vi "Signaling Events.vi"(0 "phase voltage spectra":T2(array[cluster]), 1 "signaling frequency (216.66 Hz)":dbl=216.66, 2 "reset? (F)":bool, 5 "current spectra":T2(array[cluster]), 7 "signaling voltage event settings":T5={"detection threshold [%]"=0.3, "start logical 1 length [s]"=2.99, "start logical 0 length [s]"=2.33, "maximum event length [s]"=64.0}, 9 "system info in":refnum<class "EP System Info.lvclass">, 11 "error in (no error)":errorcluster, 12 "timestamp":timestamp, 13 "interval length [s]":dbl=0.2) -> (4 "signaling voltage events":T4(array[cluster]), 10 "system info out":refnum<class "EP System Info.lvclass">, 15 "error out":errorcluster)   [LabVIEW 2014, in "NI_EP_Power Quality.lvlib"]
doc: "Detects signaling voltage events in a voltage spectrum.\n\nThis VI supports measuring single-bus single-line or multiple-bus single-line systems."
uses:
  <vilib>/addons/Electrical Power/PQ/NI_EP_Power Quality.lvlib
  <vilib>/addons/Electrical Power/PQ/Common/Controls/ep_AI Data Channel.ctl
  <vilib>/addons/Electrical Power/PQ/Common/Controls/ep_Phase.ctl
  <vilib>/addons/Electrical Power/PQ/Common/Classes/System Info/EP System Info.lvclass
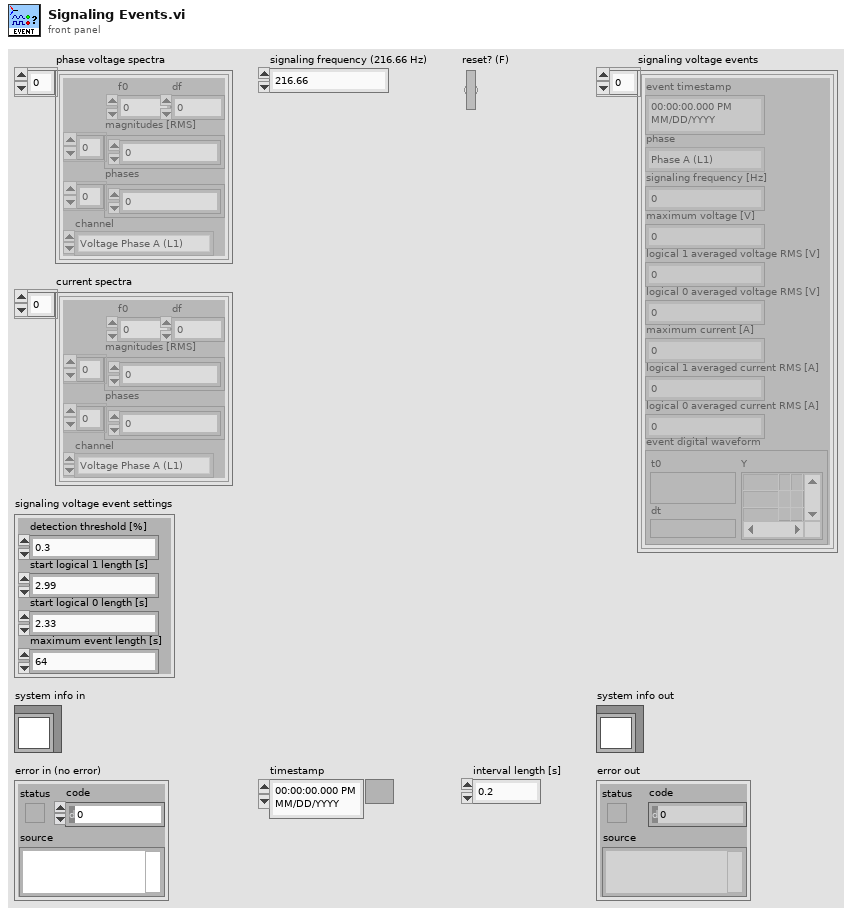
[diagram p1: front panel]
types:
  T1 = typedef "NI_EP_Power Quality.lvlib/ep_AI Data Channel.ctl" = enum16{"Voltage Phase A (L1)", "Voltage Phase B (L2)", "Voltage Phase C (L3)", "Voltage Phase N (Neutral)", "Current Phase A (L1)", "Current Phase B (L2)", "Current Phase C (L3)", "Current Phase N (Neutral)"}
  T2 = cluster{"f0":dbl, "df":dbl, "magnitudes [RMS]":dbl[], "phases":dbl[], "channel":T1}[]
  T3 = typedef "NI_EP_Power Quality.lvlib/ep_Phase.ctl" = enum16{"Phase A (L1)", "Phase B (L2)", "Phase C (L3)", "Phase N", "~3 Phases"}
  T4 = cluster{"event timestamp":timestamp, "phase":T3, "signaling frequency [Hz]":dbl, "maximum voltage [V]":dbl, "logical 1 averaged voltage RMS [V]":dbl, "logical 0 averaged voltage RMS [V]":dbl, "maximum current [A]":dbl, "logical 1 averaged current RMS [A]":dbl, "logical 0 averaged current RMS [A]":dbl, "event digital waveform":digitalwaveform}[]
  T5 = cluster{"detection threshold [%]":dbl, "start logical 1 length [s]":dbl, "start logical 0 length [s]":dbl, "maximum event length [s]":dbl}
  T6 = cluster{"f0":dbl, "df":dbl, "magnitudes [RMS]":dbl[], "phases":dbl[], "channel":T1}
  T7 = cluster{"event time":timestamp, "phase":T3, "signaling frequency [Hz]":dbl, "event voltage max. [V]":dbl, "event voltage log. 1 [V]":dbl, "event voltage log. 0 [V]":dbl, "event current max. [A]":dbl, "event current log. 1 [A]":dbl, "event current log. 0 [A]":dbl, "event digital waveform":digitalwaveform}
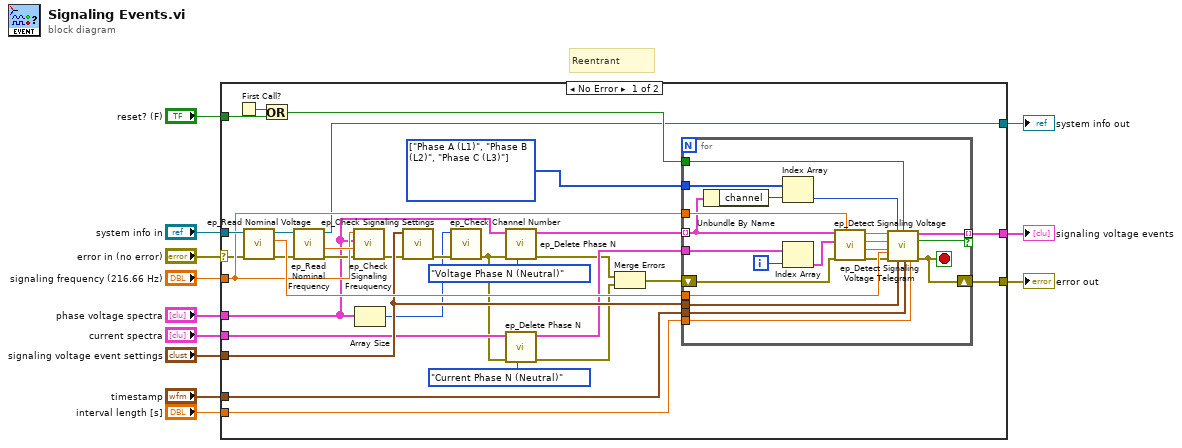
[diagram p0: block diagram]
diagram:
  # "Reentrant"
  n1 = case shown="No Error" "error in (no error)" {
    selector: "error in (no error)" -> [w32 w65]
    tunnel: "system info in" -> [w43 w66]
    tunnel: "current spectra" -> [w19 _]
    tunnel: [w22 w66] -> w10
    tunnel: "timestamp" -> [w20 _]
    tunnel: "interval length [s]" -> [w39 _]
    tunnel: "reset? (F)" -> [w37 _]
    tunnel: "phase voltage spectra" -> [w23 _]
    tunnel: "signaling frequency (216.66 Hz)" -> [w34 _]
    tunnel: [w29 w65] -> w4
    tunnel: "signaling voltage event settings" -> [w33 _]
    tunnel: [w28 _] -> w1
    frame No Error {
      w27 = T3[] [enum."Phase A (L1)", enum."Phase B (L2)", enum."Phase C (L3)"] items=["Phase A (L1)", "Phase B (L2)", "Phase C (L3)", "Phase N", "~3 Phases"]
      n2 = First Call?() -> (First Call?: T/F=w38:bool)
      n3 = call <vilib>:"ep_Read Nominal Voltage.vi"("error in (no error)"=w32, "system info in"=w43) -> ("error out"=w40:errorcluster, "nominal voltage [V]"=w42:dbl, "system info out"=w41:refnum<class "EP System Info.lvclass">)  [unwired: 7 in]
      n4 = Or(x=w38, y=w37) -> (x .or. y?=w36:bool)
      n5 = call <vilib>:"ep_Read Nominal Frequency.vi"("error in (no error)"=w40, "system info in"=w41) -> ("error out"=w31:errorcluster, "nominal frequency value"=w35:dbl, "system info out"=w22:refnum<class "EP System Info.lvclass">)  [unwired: 6 in, 1 out]
      n6 = call <vilib>:"ep_Check Signaling Freuquency.vi"("error in (no error)"=w31, "nominal frequency value"=w35, "phase voltage spectra"=w23, "signaling frequency [Hz]"=w34) -> ("error out"=w30:errorcluster)  [unwired: 7 in]
      n7 = Array Size(array=w23) -> (size(s)=w24:i32)
      n8 = call <vilib>:"ep_Check Signaling Settings.vi"("error in (no error)"=w30, "signaling voltage event settings"=w33) -> ("error out"=w25:errorcluster)  [unwired: 9 in]
      n9 = call <vilib>:"ep_Check Channel Number.vi"("channel number"=w24, "error in (no error)"=w25) -> ("error out"=w18:errorcluster)  [unwired: 13 in]
      n10 = call <vilib>:"ep_Delete Phase N.vi"("channel"=ep_AI_Data_Channel."Voltage Phase N (Neutral)", "error in (no error)"=w18, "spectra in"=w23) -> ("error out"=w14:errorcluster, "spectra out"=w26:T2)  [unwired: 7 in]
      n11 = call <vilib>:"ep_Delete Phase N.vi"("channel"=ep_AI_Data_Channel."Current Phase N (Neutral)", "error in (no error)"=w18, "spectra in"=w19) -> ("error out"=w13:errorcluster, "spectra out"=w16:T2)  [unwired: 7 in]
      n12 = Merge Errors(w14, w13) -> (w15:errorcluster)
      n13 = for {
        tunnel: w42 -> [w64]
        tunnel: w20 -> [w63]
        tunnel: w39 -> [w62]
        tunnel: w36 -> [w61]
        tunnel: w34 -> [w60]
        tunnel: w33 -> [w59]
        tunnel: [w58] -> w28 mode=indexing if=w50
        tunnel: w16 -> [w56]
        tunnel: w26 -> [w47] mode=indexing
        shift-right: [w48] -> w29
        shift-left: w15 -> [w57]
        tunnel: w27 -> [w46]
        i -> [w49]
        stop <- w48 stop-if-true
        n14 = Unbundle By Name(w47) -> ("channel"=w45:T1)
        n15 = Index Array(array=w46, index=w45) -> (element=w44:T3)
        n16 = Index Array(array=w56, index=w49) -> (element=w55:T6)
        n17 = call <vilib>:"ep_Detect Signaling Voltage.vi"("signaling frequency"=w60, "error in (no error)"=w57, "current spectrum (5Hz step)"=w55, "voltage spectrum (5Hz step)"=w47) -> ("error out"=w51:errorcluster, "detected signaling frequency [Hz]"=w52:dbl, "signaling current RMS [A]"=w53:dbl, "signaling voltage RMS [V]"=w54:dbl)  [unwired: 4 in]
        n18 = call <vilib>:"ep_Detect Signaling Voltage Telegram.vi"("signaling voltage RMS [V]"=w54, "phase"=w44, "restart? (F)"=w61, "signaling current RMS [A]"=w53, "detected signaling frequency [Hz]"=w52, "nominal voltage [V]"=w64, "signaling voltage event settings"=w59, "time stamp"=w63, "interval length [sec]"=w62, "error in (no error)"=w51) -> ("Telegram"=w58:T7, "data valid?"=w50:bool, "error out"=w48:errorcluster)  [unwired: 3 in]
      }
    }
    frame Error {
    }
  }
  "error out" <- w4
  "signaling voltage events" <- w1
  "system info out" <- w10
